vi "Init.vi"(8 "error in (no error)":errorcluster, 11 "Text Report in":refnum<class "Text Report.lvclass">) -> (0 "error out":errorcluster, 3 "Text Report out":refnum<class "Text Report.lvclass">)   [LabVIEW 2020, in "Text Report.lvclass"]
uses:
  Text Report.lvclass
  Text Report.lvclass/Text Report.ctl
  <vilib>/Utility/sysdir.llb/Get System Directory.vi
  <vilib>/Utility/libraryn.llb/Create Directory Recursive.vi
  User Interface/Support/Paths.lvlib
  Framework/Configuration Manager/Configuration Manager.lvclass
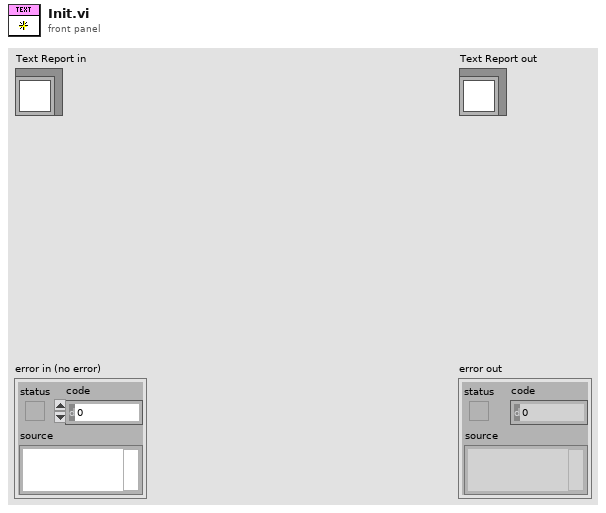
[diagram p1: front panel]
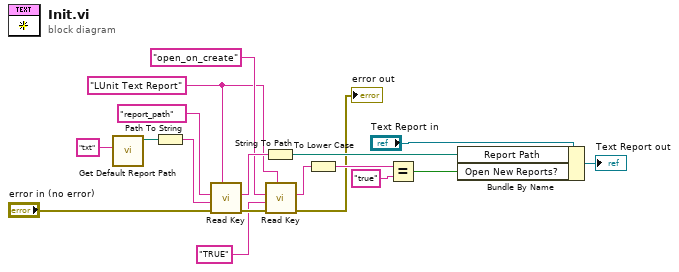
[diagram p0: block diagram]
diagram:
  w11 = "LUnit Text Report"
  n1 = call "Get Default Report Path.vi"("File Extension"="txt") -> ("Default Report Path"=w9:path)  [unwired: 9 in, 1 out]
  n2 = Path To String(path=w9) -> (string=w8:string)
  n3 = call "Read Key.vi"("section"=w11, "error in (no error)"="error in (no error)", "default value"=w8, "key"="report_path" ("Name")) -> ("error out"=w18:errorcluster, "value"=w16:string)  [unwired: 6 in]
  n4 = String To Path(string=w16) -> (path=w7:path)
  n5 = call "Read Key.vi"("section"=w11, "error in (no error)"=w18, "default value"="TRUE", "key"="open_on_create" ("Name")) -> ("error out"=→"error out":errorcluster, "value"=w14:string)  [unwired: 6 in]
  n6 = To Lower Case(string=w14) -> (all lower case string=w13:string)
  n7 = Equal?(x=w13, y="true") -> (x = y?=w6:bool)
  n8 = Bundle By Name(cluster="Text Report in", "Report Path"=w7, "Open New Reports?"=w6) -> (→"Text Report out":refnum<class "Text Report.lvclass">)
